vi "Remove Points.vi"(8 "error in (no error)":errorcluster, 10 "point_ids":u32[](array[numeric]), 11 "KD Tree in":refnum<class "KD Tree.lvclass">) -> (0 "error out":errorcluster, 3 "KD Tree out":refnum<class "KD Tree.lvclass">)   [LabVIEW 2020, in "KD Tree.lvlib" / "KD Tree.lvclass"]
uses:
  KD Tree.lvclass
  KD Tree.lvlib
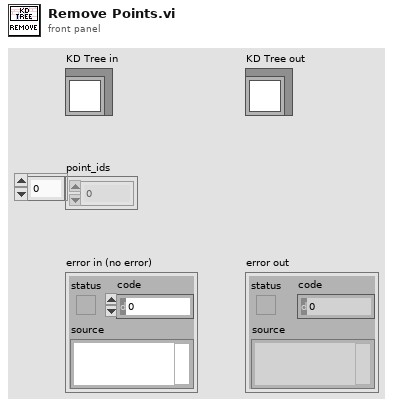
[diagram p1: front panel]
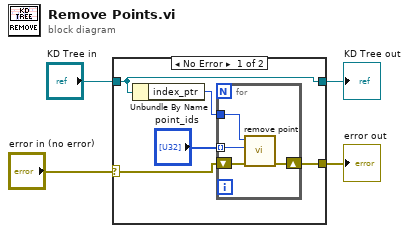
[diagram p0: block diagram]
diagram:
  n1 = case shown="No Error" "error in (no error)" {
    selector: "error in (no error)" -> [w6 w15]
    tunnel: [w5 w15] -> w3
    tunnel: [w9 w14] -> w1
    tunnel: "KD Tree in" -> [w9 w14]
    frame No Error {
      n2 = Unbundle By Name(w9) -> ("index_ptr"=w8:u64)
      n3 = for {
        tunnel: w8 -> [w13]
        tunnel: "point_ids" -> [w12] mode=indexing
        shift-right: [w10] -> w5
        shift-left: w6 -> [w11]
        n4 = call "remove point.vi"("error in (no error)"=w11, "point_id"=w12, "index_ptr"=w13) -> ("error out"=w10:errorcluster)  [unwired: 7 in, 1 out]
      }
    }
    frame Error {
    }
  }
  "error out" <- w3
  "KD Tree out" <- w1
